vi "NearWaypointTest.vi"(6 "Capture Radius":dbl=10.0, 8 "X (Current)":dbl, 9 "Y (Current)":dbl, 10 "X (Waypoint)":dbl, 11 "Y (Waypoint)":dbl) -> (2 "AtWaypoint":bool)   [LabVIEW 2011]
doc: "This VI checks to see if the robots curretn position is close to the next waypoint. If it is, it sets a boolean flag to allow a case statement to update the MDF"
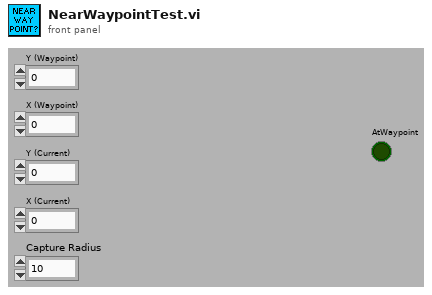
[diagram p1: front panel]
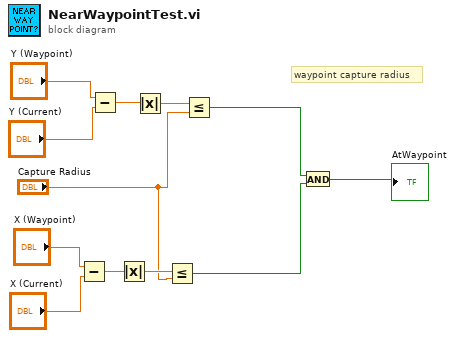
[diagram p0: block diagram]
diagram:
  # "waypoint capture radius"
  n1 = Subtract(x="X (Waypoint)", y="X (Current)") -> (x-y=w7:dbl)
  n2 = Subtract(x="Y (Waypoint)", y="Y (Current)") -> (x-y=w8:dbl)
  n3 = Absolute Value(x=w7) -> (abs(x)=w6:dbl)
  n4 = Absolute Value(x=w8) -> (abs(x)=w5:dbl)
  n5 = Less Or Equal?(x=w6, y="Capture Radius") -> (x <= y?=w2:bool)
  n6 = Less Or Equal?(x=w5, y="Capture Radius") -> (x <= y?=w3:bool)
  n7 = And(x=w3, y=w2) -> (x .and. y?=→"AtWaypoint":bool)
